vi "FindBlock.vi"(7 "Start pos":dbl[](array[numeric]), 8 "Block Array in":dbl[][](array[numeric]), 9 "Robot pos":dbl[](array[numeric]), 10 "World Y array":dbl[](array[numeric]), 11 "World X array":dbl[](array[numeric])) -> (1 "ODM Global Lidar Fix Map":cluster{dbl[], dbl[]}[](graph), 2 "ASCII Block":string[](array[string]), 3 "Block Array out":dbl[][](array[numeric]))   [LabVIEW 2018]
panel:
  out "Global Line Map":cluster{dbl[], dbl[]}[](graph)
  out "Line Array":dbl[][][](array[numeric])
  out "Line Array Size":i32[](array[numeric])
  out "Wall Seg Array":dbl[][][](array[numeric])
  out "Wall Array size":i32[](array[numeric])
  # "BX,BY,X,Y下顏色,上顏色"
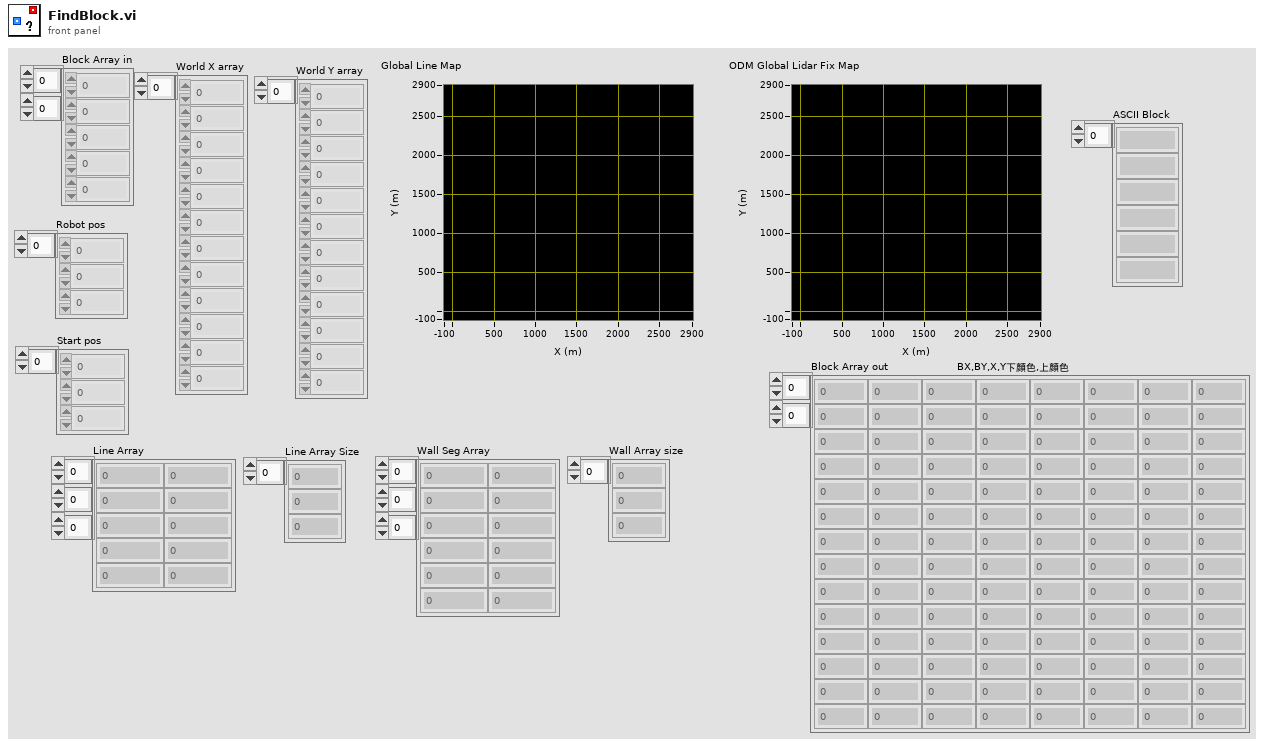
[diagram p1: front panel]
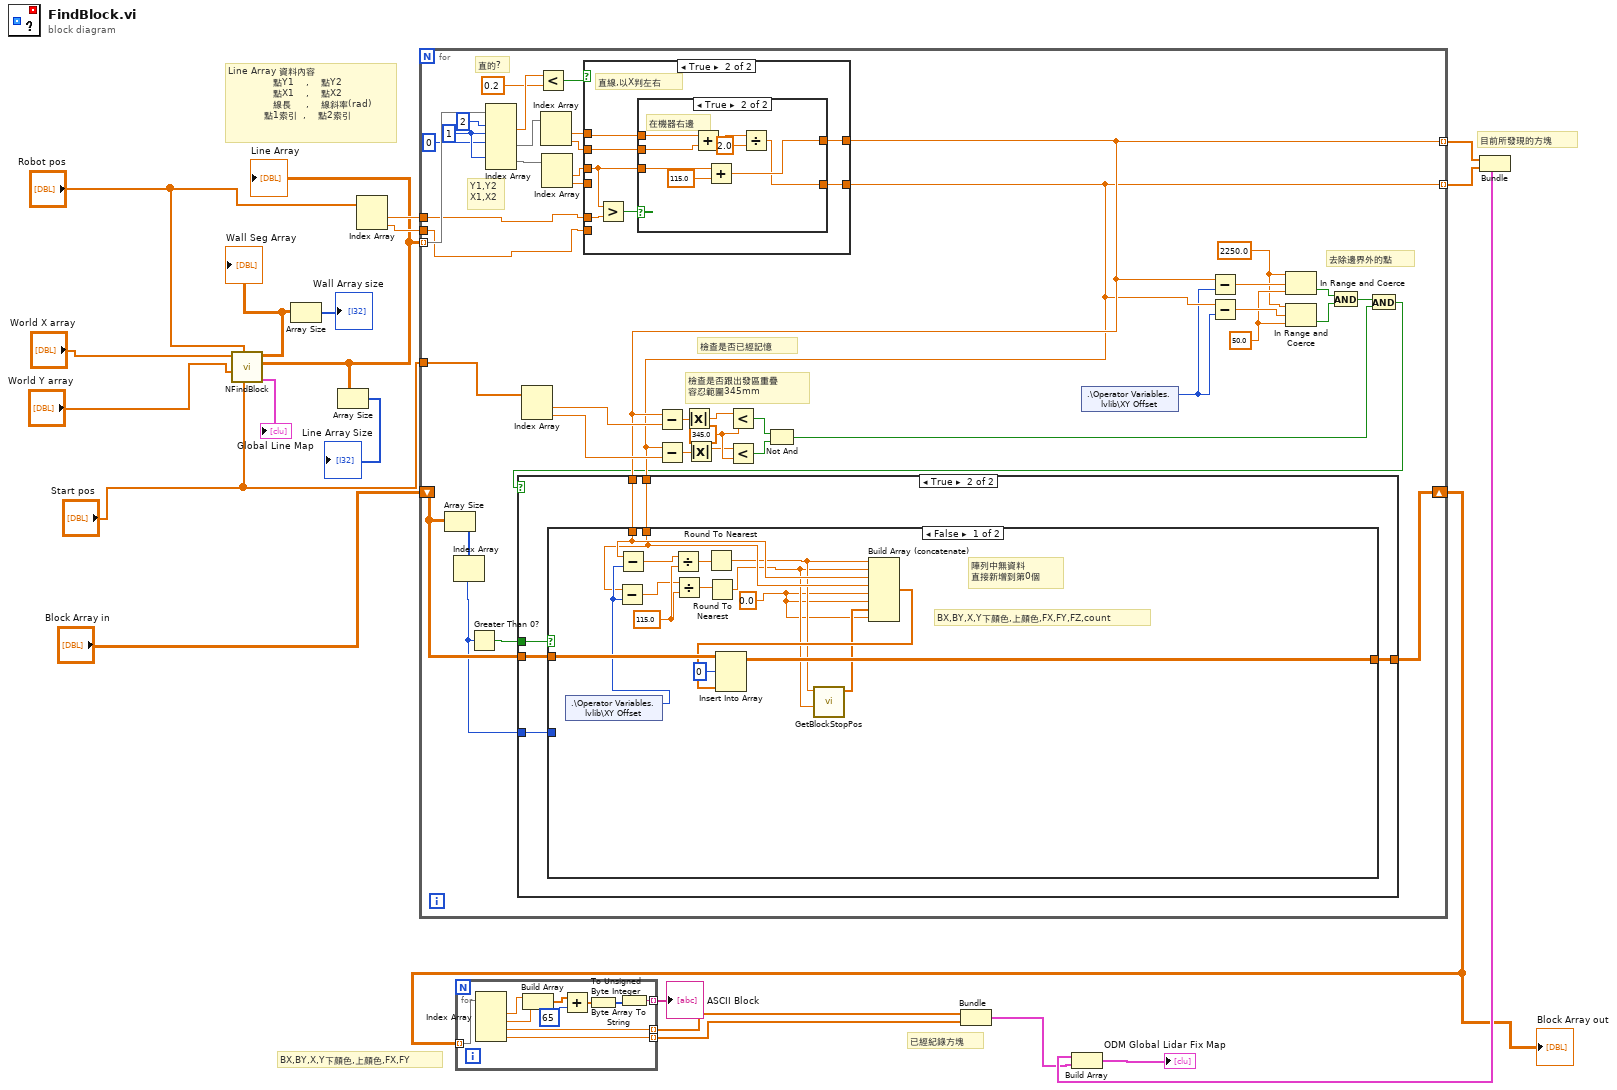
[diagram p0: block diagram]
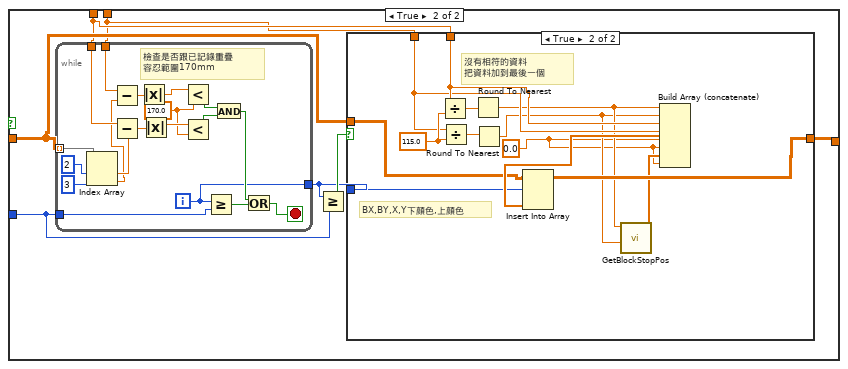
[diagram p3: hidden frame]
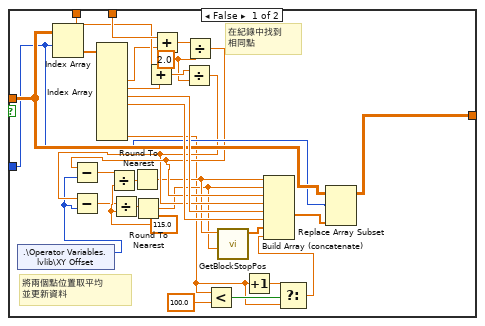
[diagram p4: hidden frame]
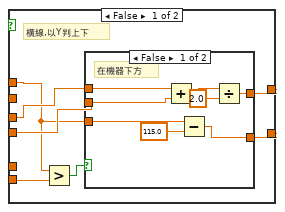
[diagram p5: hidden frame]
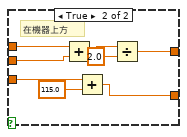
[diagram p6: hidden frame]
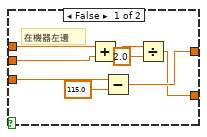
[diagram p7: hidden frame]
diagram:
  # "已經紀錄方塊"
  # "目前所發現的方塊"
  # "Line Array 資料內容\n               點Y1    ,    點Y2    \n               點X1    ,    點X2\n               線長     ,    線斜率(rad)\n            點1索引  ,    點2索引"
  # "BX,BY,X,Y下顏色,上顏色,FX,FY"
  n1 = call "NFindBlock.vi"("Start pos"="Start pos", "Robot pos"="Robot pos", "Y array"="World Y array", "X array"="World X array") -> ("Group Lidar Map"=→"Global Line Map":cluster{dbl[], dbl[]}[], "Line Array"=w3:dbl[][][], "Empty Array"=w4:dbl[][][])  [unwired: 5 in]
  "Line Array" <- w3
  "Wall Seg Array" <- w4
  n2 = Array Size(array=w4) -> (size(s)=→"Wall Array size":i32[])
  n3 = Array Size(array=w3) -> (size(s)=→"Line Array Size":i32[])
  n4 = Index Array(array="Robot pos") -> (element #1=w19:dbl, element #2=w18:dbl)  [unwired: 2 in]
  n5 = for {
    tunnel: w3 -> [w63] mode=indexing
    tunnel: w19 -> [w50]
    tunnel: w18 -> [w49]
    tunnel: [w33] -> w15 mode=indexing
    tunnel: [w32] -> w14 mode=indexing
    shift-right: [w44] -> w13
    shift-left: "Block Array in" -> [w47]
    tunnel: "Start pos" -> [w34]
    w28 = 50.0 ("upper limit")
    w27 = 2250.0 ("upper limit")
    w43 = 345.0
    w58 = 1 ("disabled index (col)")
    # "去除邊界外的點"
    # "檢查是否跟出發區重疊\n容忍範圍345mm"
    # "檢查是否已經記憶"
    # "Y1,Y2\nX1,X2"
    # "直的?"
    n6 = Array Size(array=w47) -> (size(s)=w48:i32[])
    n7 = Index Array(array=w48) -> (element=w45:i32)  [unwired: 1 in]
    n8 = Greater Than 0?(x=w45) -> (x > 0?=w46:bool)
    n9 = Index Array(array=w63, index (row) #1=2 ("index (row)"), index (col) #1=w58, index (row) #2=0 ("index (row)"), index (row) #3=w58) -> (element #1=w61:dbl, element #2=w55:dbl[], element #3=w56:dbl[])  [unwired: 2 in]
    n10 = Index Array(array=w34) -> (element #1=w38:dbl, element #2=w37:dbl)  [unwired: 2 in]
    n11 = Less?(x=w61, y=0.2) -> (x < y?=w59:bool)
    n12 = Index Array(array=w55) -> (element #1=w54:dbl, element #2=w53:dbl)  [unwired: 2 in]
    n13 = Index Array(array=w56) -> (element #1=w52:dbl, element #2=w51:dbl)  [unwired: 2 in]
    n14 = case shown="True" w59 {
      tunnel: w50 -> [_ w185]
      tunnel: w49 -> [w162 _]
      tunnel: w54 -> [w158 w182]
      tunnel: w53 -> [_ w181]
      tunnel: w52 -> [w160 w183]
      tunnel: w51 -> [w159 _]
      tunnel: [w157 w180] -> w33
      tunnel: [w156 w179] -> w32
      frame False {
        # "橫線,以Y判上下"
        n15 = Greater?(x=w158, y=w162) -> (0:w161:bool)
        n16 = case shown="False" w161 {
          tunnel: w158 -> [w167 w178]
          tunnel: w160 -> [w165 w176]
          tunnel: w159 -> [w166 w175]
          tunnel: [w164 w172] -> w157
          tunnel: [w163 w171] -> w156
          frame False {
            # "在機器下方"
            n17 = Add(x=w165, y=w166) -> (x+y=w169:dbl)
            n18 = Subtract(x=w167, y=115.0) -> (x-y=w163:dbl)
            n19 = Divide(x=w169, y=2.0) -> (x/y=w164:dbl)
          }
          frame True {
            # "在機器上方"
            n20 = Add(x=w176, y=w175) -> (x+y=w174:dbl)
            n21 = Add(x=w178, y=115.0) -> (x+y=w171:dbl)
            n22 = Divide(x=w174, y=2.0) -> (x/y=w172:dbl)
          }
        }
      }
      frame True {
        # "直線,以X判左右"
        n23 = Greater?(x=w183, y=w185) -> (0:w184:bool)
        n24 = case shown="True" w184 {
          tunnel: w183 -> [w190 w201]
          tunnel: w182 -> [w188 w199]
          tunnel: w181 -> [w189 w198]
          tunnel: [w187 w195] -> w180
          tunnel: [w186 w194] -> w179
          frame False {
            # "在機器左邊"
            n25 = Add(x=w188, y=w189) -> (x+y=w192:dbl)
            n26 = Subtract(x=w190, y=115.0) -> (x-y=w187:dbl)
            n27 = Divide(x=w192, y=2.0) -> (x/y=w186:dbl)
          }
          frame True {
            # "在機器右邊"
            n28 = Add(x=w199, y=w198) -> (x+y=w197:dbl)
            n29 = Add(x=w201, y=115.0) -> (x+y=w195:dbl)
            n30 = Divide(x=w197, y=2.0) -> (x/y=w194:dbl)
          }
        }
      }
    }
    n31 = Subtract(x=w33, y=w38) -> (x-y=w39:dbl)
    n32 = Subtract(x=w32, y=w37) -> (x-y=w40:dbl)
    n33 = Absolute Value(x=w39) -> (abs(x)=w41:dbl)
    n34 = Absolute Value(x=w40) -> (abs(x)=w42:dbl)
    n35 = Less?(x=w41, y=w43) -> (x < y?=w36:bool)
    n36 = Less?(x=w42, y=w43) -> (x < y?=w35:bool)
    n37 = Not And(1:w35, 2:w36) -> (0:w23:bool)
    n38 = shared-variable ".\\Operator Variables.lvlib\\XY Offset"() -> (w31:i16)  [unwired: 1 in, 1 out]
    n39 = Subtract(x=w33, y=w31) -> (x-y=w30:dbl)
    n40 = Subtract(x=w32, y=w31) -> (x-y=w29:dbl)
    n41 = In Range and Coerce(upper limit=w27, x=w30, lower limit=w28) -> (In Range?=w25:bool)  [unwired: 1 out]
    n42 = In Range and Coerce(upper limit=w27, x=w29, lower limit=w28) -> (In Range?=w26:bool)  [unwired: 1 out]
    n43 = And(x=w25, y=w26) -> (x .and. y?=w24:bool)
    n44 = And(x=w24, y=w23) -> (x .and. y?=w22:bool)
    n45 = case shown="True" w22 {
      tunnel: w47 -> [w64 w70]
      tunnel: w46 -> [_ w69]
      tunnel: w45 -> [_ w68]
      tunnel: [w64 w67] -> w44
      tunnel: w33 -> [_ w66]
      tunnel: w32 -> [_ w65]
      frame False {
      }
      frame True {
        n46 = case shown="False" w69 {
          tunnel: w66 -> [w78 w89]
          tunnel: w65 -> [w75 w88]
          tunnel: w70 -> [w83 w91]
          tunnel: [w80 w87] -> w67
          tunnel: w68 -> [_ w93]
          frame False {
            w71 = 0.0
            w86 = 115.0
            # "BX,BY,X,Y下顏色,上顏色,FX,FY,FZ,count"
            # "陣列中無資料\n直接新增到第0個"
            n47 = shared-variable ".\\Operator Variables.lvlib\\XY Offset"() -> (w79:i16)  [unwired: 1 in, 1 out]
            n48 = Subtract(x=w75, y=w79) -> (x-y=w76:dbl)
            n49 = Subtract(x=w78, y=w79) -> (x-y=w77:dbl)
            n50 = Divide(x=w77, y=w86) -> (x/y=w85:dbl)
            n51 = Divide(x=w76, y=w86) -> (x/y=w84:dbl)
            n52 = Round To Nearest(number=w85) -> (nearest integer value=w74:dbl)
            n53 = Round To Nearest(number=w84) -> (nearest integer value=w73:dbl)
            n54 = call "GetBlockStopPos.vi"("YB"=w73, "XB"=w74) -> ("Array"=w72:dbl[])  [unwired: 8 in, 1 out]
            n55 = Build Array (concatenate)(w74, w73, w78, w75, w71, w71, w72, w71) -> (w82:dbl[])
            n56 = Insert Into Array(array=w83, index (row)=0, new element=w82) -> (w80:dbl[][])  [unwired: 1 in]
          }
          frame True {
            n57 = while {
              tunnel: w89 -> [w153]
              tunnel: w88 -> [w152]
              tunnel: w91 -> [w155] mode=indexing
              tunnel: w93 -> [w141]
              tunnel: [w138] -> w90
              i -> [w138]
              stop <- w137 stop-if-true
              w144 = 170.0
              # "檢查是否跟已記錄重疊\n容忍範圍170mm"
              n58 = Index Array(array=w155, index #1=2 ("index"), index #2=3 ("index")) -> (element #1=w154:dbl, element #2=w151:dbl)
              n59 = Subtract(x=w152, y=w151) -> (x-y=w148:dbl)
              n60 = Subtract(x=w153, y=w154) -> (x-y=w147:dbl)
              n61 = Absolute Value(x=w148) -> (abs(x)=w146:dbl)
              n62 = Absolute Value(x=w147) -> (abs(x)=w145:dbl)
              n63 = Less?(x=w146, y=w144) -> (x < y?=w142:bool)
              n64 = Less?(x=w145, y=w144) -> (x < y?=w143:bool)
              n65 = Greater Or Equal?(x=w138, y=w141) -> (x >= y?=w140:bool)
              n66 = And(x=w142, y=w143) -> (x .and. y?=w139:bool)
              n67 = Or(x=w139, y=w140) -> (x .or. y?=w137:bool)
            }
            n68 = Greater Or Equal?(x=w90, y=w93) -> (x >= y?=w92:bool)
            n69 = case shown="True" w92 {
              tunnel: w91 -> [w118 w132]
              tunnel: w90 -> [w107 w131]
              tunnel: w89 -> [w115 w130]
              tunnel: w88 -> [w114 w129]
              tunnel: [w116 w128] -> w87
              frame False {
                w108 = 115.0
                w109 = 2.0 ("y")
                # "在紀錄中找到\n相同點"
                # "將兩個點位置取平均\n並更新資料"
                n70 = shared-variable ".\\Operator Variables.lvlib\\XY Offset"() -> (w102:i16)  [unwired: 1 in, 1 out]
                n71 = Index Array(array=w118, index (row)=w107) -> (element=w121:dbl[])  [unwired: 1 in]
                n72 = Index Array(array=w121) -> (element #3=w113:dbl, element #4=w112:dbl, element #5=w120:dbl, element #6=w119:dbl, element #10=w94:dbl)  [unwired: 10 in, 5 out]
                n73 = Add(x=w114, y=w112) -> (x+y=w110:dbl)
                n74 = Add(x=w115, y=w113) -> (x+y=w111:dbl)
                n75 = Divide(x=w110, y=w109) -> (x/y=w104:dbl)
                n76 = Subtract(x=w104, y=w102) -> (x-y=w103:dbl)
                n77 = Divide(x=w103, y=w108) -> (x/y=w122:dbl)
                n78 = Round To Nearest(number=w122) -> (nearest integer value=w100:dbl)
                n79 = Divide(x=w111, y=w109) -> (x/y=w106:dbl)
                n80 = Subtract(x=w106, y=w102) -> (x-y=w105:dbl)
                n81 = Divide(x=w105, y=w108) -> (x/y=w123:dbl)
                n82 = Round To Nearest(number=w123) -> (nearest integer value=w101:dbl)
                n83 = Less?(x=w94, y=100.0) -> (x < y?=w97:bool)
                n84 = call "GetBlockStopPos.vi"("YB"=w100, "XB"=w101) -> ("Array"=w99:dbl[])  [unwired: 8 in, 1 out]
                n85 = Increment(x=w94) -> (x+1=w96:dbl)
                n86 = Select(t=w96, s=w97, f=w94) -> (s? t:f=w95:dbl)
                n87 = Build Array (concatenate)(w101, w100, w106, w104, w120, w119, w99, w95) -> (w117:dbl[])
                n88 = Replace Array Subset(array=w118, new element=w117, index (row)=w107) -> (w116:dbl[][])  [unwired: 1 in]
              }
              frame True {
                w124 = 0.0
                w136 = 115.0
                # "BX,BY,X,Y下顏色,上顏色"
                # "沒有相符的資料\n把資料加到最後一個"
                n89 = Divide(x=w130, y=w136) -> (x/y=w135:dbl)
                n90 = Divide(x=w129, y=w136) -> (x/y=w134:dbl)
                n91 = Round To Nearest(number=w135) -> (nearest integer value=w127:dbl)
                n92 = Round To Nearest(number=w134) -> (nearest integer value=w126:dbl)
                n93 = call "GetBlockStopPos.vi"("YB"=w126, "XB"=w127) -> ("Array"=w125:dbl[])  [unwired: 8 in, 1 out]
                n94 = Build Array (concatenate)(w127, w126, w130, w129, w124, w124, w125, w124) -> (w133:dbl[])
                n95 = Insert Into Array(array=w132, index (row)=w131, new element=w133) -> (w128:dbl[][])  [unwired: 1 in]
              }
            }
          }
        }
      }
    }
  }
  "Block Array out" <- w13
  n96 = for {
    tunnel: w13 -> [w211] mode=indexing
    tunnel: [w210] -> w12 mode=indexing
    tunnel: [w209] -> w11 mode=indexing
    tunnel: [w202] -> w9 mode=indexing
    n97 = Index Array(array=w211) -> (element #1=w208:dbl, element #2=w207:dbl, element #3=w210:dbl, element #4=w209:dbl)  [unwired: 4 in]
    n98 = Build Array(w208, w207) -> (w206:dbl[])
    n99 = Add(x=w206, y=65) -> (x+y=w204:dbl[])
    n100 = To Unsigned Byte Integer(number=w204) -> (unsigned 8bit integer=w203:u8[])
    n101 = Byte Array To String(unsigned byte array=w203) -> (string=w202:string)
  }
  "ASCII Block" <- w9
  n102 = Bundle(w12, w11) -> (w10:cluster{dbl[], dbl[]})  [unwired: 1 in]
  n103 = Bundle(w15, w14) -> (w17:cluster{dbl[], dbl[]})  [unwired: 1 in]
  n104 = Build Array(w17, w10) -> (→"ODM Global Lidar Fix Map":cluster{dbl[], dbl[]}[])
